vi "Demo-Metrics_Viz.vi"() -> ()   [LabVIEW 2020]
uses:
  <vilib>/Utility/miscctls.llb/LVRectTypeDef.ctl
  <vilib>/UPVI/lvhdf5/group.llb/H5G_obj_t.ctl
  <vilib>/UPVI/lvhdf5/file.llb/LVH5F Operation.ctl
  <vilib>/UPVI/lvhdf5/dataset.llb/LVH5D Operation.ctl
  <vilib>/UPVI/lvhdf5/file.llb/H5Fopen.vi
  <vilib>/UPVI/lvhdf5/utility.llb/Select HDF5 Dialog.vi
  <vilib>/UPVI/lvhdf5/utility.llb/Select HDF5 Dialog (File and Object).vi
  <vilib>/UPVI/lvhdf5/dataset.llb/Simple H5Dread (Variant).vi
  <vilib>/UPVI/lvhdf5/utility.llb/Select HDF5 Dialog (Object Only).vi
  <vilib>/UPVI/lvhdf5/dataset.llb/Simple H5Dread.xnode
  <vilib>/UPVI/lvhdf5/library.llb/HDF5 Ref.ctl
  <vilib>/UPVI/lvhdf5/library.llb/HDF5 Ref.lvclass
  <vilib>/UPVI/lvhdf5/file.llb/H5Fclose.vi
  <vilib>/UPVI/lvhdf5/identifier.llb/Not an HDF5 Refnum Constant.vi
  <vilib>/UPVI/lvhdf5/dataset.llb/OpenCreateReplace Dataset.vi
  <vilib>/UPVI/lvhdf5/dataset.llb/H5Dget_space.vi
  <vilib>/UPVI/lvhdf5/dataspace.llb/H5Sget_simple_extent_dims.vi
  <vilib>/UPVI/lvhdf5/dataspace.llb/H5Sselect_hyperslab.vi
  <vilib>/UPVI/lvhdf5/dataset.llb/H5Dread (Variant).vi
  <vilib>/UPVI/lvhdf5/attribute.llb/private/LVH5AreadWDTAttrs.vi
  <vilib>/UPVI/lvhdf5/dataspace.llb/H5Sclose.vi
  <vilib>/Utility/error.llb/Error Cluster From Error Code.vi
  <vilib>/UPVI/lvhdf5/dataset.llb/H5Dclose.vi
panel:
  out "Metrics Plot":cluster{u64[], "Data out":dbl[]}(graph)
  in  "HDF5 Path or Ref":path=path "T:/2022-07-19/Net15 Nucleo H7 Photodiode-2022-07-19_23h15m22s994ms.h5"
  # "Simple Demo of Metrics Visualization from an Existing HDF5 File"
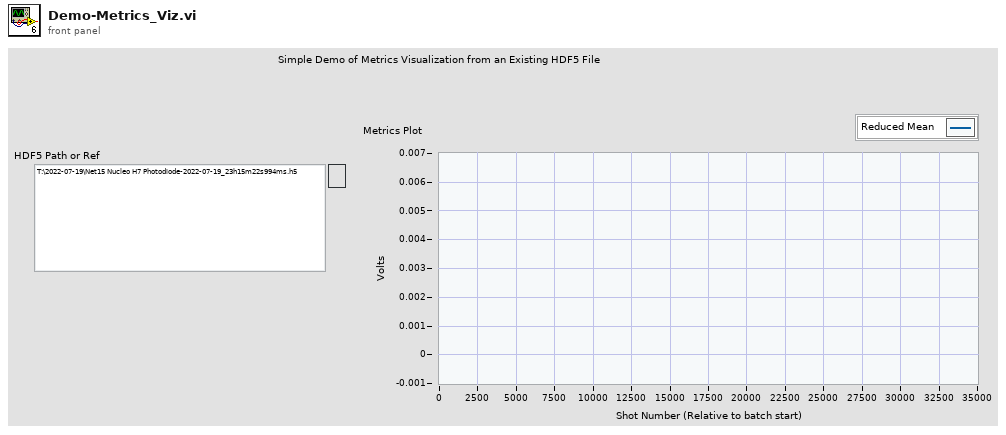
[diagram p1: front panel]
types:
  T1 = typedef "HDF5 Ref.ctl" = refnum<class "HDF5 Ref.lvclass">
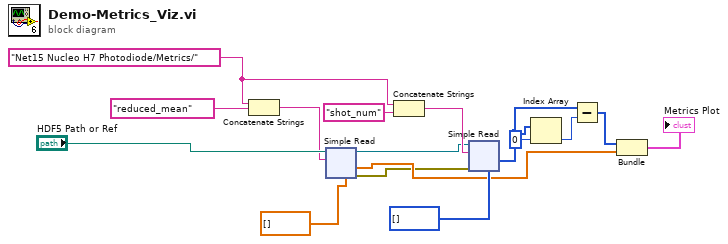
[diagram p0: block diagram]
diagram:
  w12 = "Net15 Nucleo H7 Photodiode/Metrics/"
  n1 = Concatenate Strings(w12, "reduced_mean" ("Dataset Path")) -> (w13:string)
  n2 = xnode "Simple Read"("Dataset Path"=w13, "HDF5 Path or Ref"="HDF5 Path or Ref", "Data"=dbl[] []) -> ("HDF5 Ref out"=w9:T1, "error out"=w5:errorcluster, "Data out"=w6:dbl[])  [unwired: 1 in, 1 out]
  n3 = Concatenate Strings(w12, "shot_num" ("string")) -> (w10:string)
  n4 = xnode "Simple Read"("Dataset Path"=w10, "error in (no error)"=w5, "HDF5 Path or Ref"=w9, "Data"=u64[] []) -> ("Data out"=w2:u64[])  [unwired: 3 out]
  n5 = Index Array(array=w2, index=0) -> (element=w3:u64)
  n6 = Subtract(x=w2, y=w3) -> (x-y=w1:u64[])
  n7 = Bundle(w1, "Data out"=w6) -> (→"Metrics Plot":cluster{u64[], "Data out":dbl[]})  [unwired: 1 in]
